vi "TempPreRunGraph_DP_Ver1.0.vi"(0 "T Array":dbl[](array[numeric]), 1 "Temp Display Cluster (Need RMS)":cluster{"RMS T:":dbl, "STD T:":dbl, "T":dbl} {"STD T:" format="%_5g"; "T" min=0.0 format="%_5g"; "RMS T:" format="%_5g"}, 2 "Set Pt":dbl, 3 "Delta T":dbl=0.008) -> (5 "Temp Graph":dbl[][](graph))   [LabVIEW 2012]
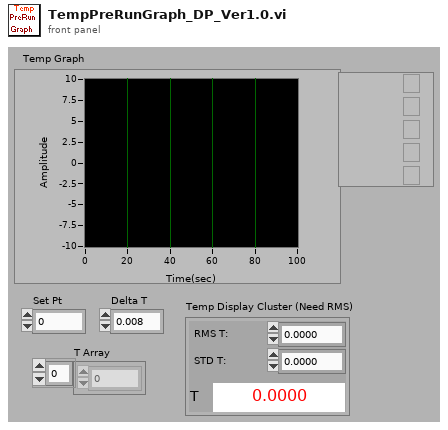
[diagram p1: front panel]
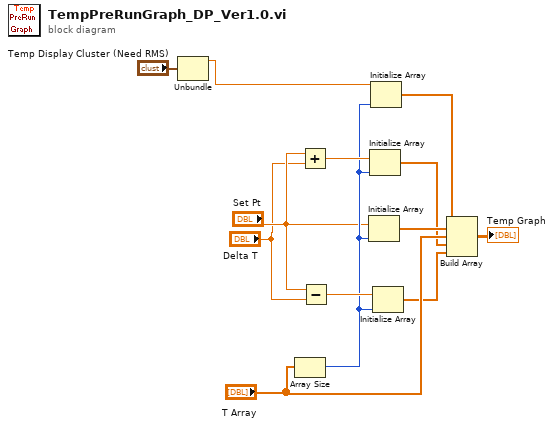
[diagram p0: block diagram]
diagram:
  n1 = Unbundle("Temp Display Cluster (Need RMS)") -> ("RMS T:"=w1:dbl)  [unwired: 2 out]
  n2 = Array Size(array="T Array") -> (size(s)=w11:i32)
  n3 = Add(x="Set Pt", y="Delta T") -> (x+y=w13:dbl)
  n4 = Subtract(x="Set Pt", y="Delta T") -> (x-y=w12:dbl)
  n5 = Initialize Array("Set Pt", w11) -> (w8:dbl[])
  n6 = Initialize Array(w13, w11) -> (w6:dbl[])
  n7 = Initialize Array(w1, w11) -> (w10:dbl[])
  n8 = Initialize Array(w12, w11) -> (w5:dbl[])
  n9 = Build Array(w10, w8, "T Array", w6, w5) -> (→"Temp Graph":dbl[][])
